vi "Keyence.File.Read.vi"(7 "log path":path, 8 "error in":errorcluster, 11 "segtings path":path) -> (0 "error out":errorcluster)   [LabVIEW 2016]
uses:
  tools/Tma.lib/nlconfig.llb/fp2ini mode.ctl
  Keyence.Global.vi
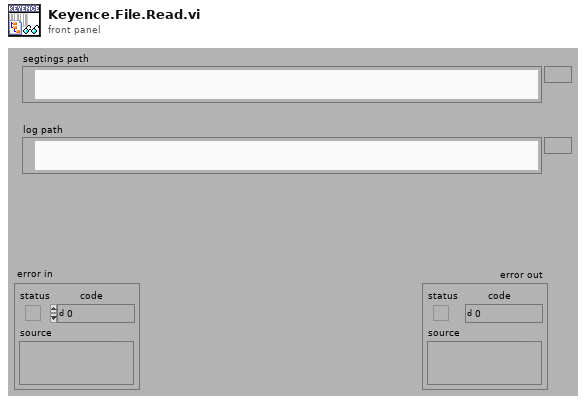
[diagram p1: front panel]
types:
  T1 = typedef "fp2ini mode.ctl" = enum16{"Read Controls", "Write Controls", "Write Indicators", "Read Indicators", "Write all", "Read all"}
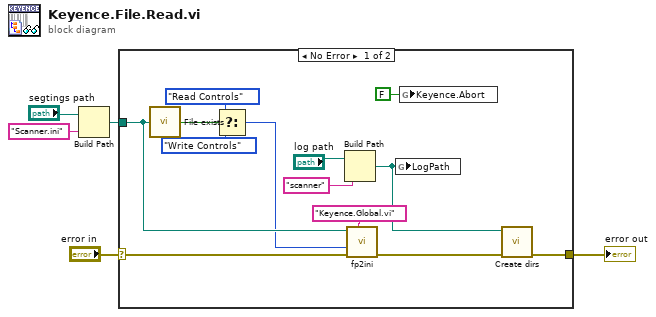
[diagram p0: block diagram]
diagram:
  n1 = Build Path(base path="segtings path", name or relative path="Scanner.ini") -> (appended path=w2:path)
  n2 = case shown="No Error" "error in" {
    selector: "error in" -> [w18 w19]
    tunnel: [w7 w19] -> w5
    tunnel: w2 -> [w17 _]
    frame No Error {
      n3 = call "File exists.vi"("file path"=w17) -> ("exists?"=w15:bool)  [unwired: 4 in]
      n4 = Select(t=fp2ini_mode."Read Controls" ("mode"), s=w15, f=fp2ini_mode."Write Controls" ("mode")) -> (s? t:f=w12:T1)
      n5 = Build Path(base path="log path", name or relative path="scanner") -> (appended path=w8:path)
      n6 = call "fp2ini.vi"("vi-name (caller if empty)"="Keyence.Global.vi", "error in"=w18, "mode"=w12, "ini-file path"=w17) -> ("error out"=w10:errorcluster)  [unwired: 3 in, 4 out]
      n7 = global write "Keyence.Global.vi" "LogPath"(w8) -> ()
      n8 = global write "Keyence.Global.vi" "Keyence.Abort"(FALSE ("Keyence.Abort")) -> ()
      n9 = call "Create dirs.vi"("error in (no error)"=w10, "deepest dir"=w8) -> ("error"=w7:errorcluster)  [unwired: 9 in]
    }
    frame Error {
    }
  }
  "error out" <- w5
